vi "GolieKick.vi"(6 "Current State":dbl=4.0, 8 "atacando contra?":bool=TRUE, 9 "balls":T1[](array[typedef])=[{"x"=-974.5169677734375, "y"=-3444.3310546875, "timestamp"=timestamp(2082759045.994995 s since 1904-01-01)}], 10 "Field Size in":T4={"line_width"=10, "field_length"=9000, "field_width"=6000, "boundary_width"=250, "referee_width"=425, "goal_width"=700, "goal_depth"=180, "goal_wall_width"=20, "center_circle_radius"=500, "defense_radius"=500, "defense_stretch"=350, "free_kick_from_defense_dist"=700, "penalty_spot_from_field_line_dist"=450, "penalty_line_from_spot_dist"=350}, 11 "Robot in":T2={"id"=5, "function"=enum."Attacker", "x"=-983.1382446289062, "y"=-3000.010498046875, "orientation"=-1.5516623258590698, "v_tangent"=0.0, "v_normal"=0.0, "v_ang"=0.0, "kick_x"=0.0, "kick_z"=0.0, "dribble"=FALSE, "Timestamp"=timestamp(2082759045.994995 s since 1904-01-01), "dest_x"=0.0, "dest_y"=0.0, "dest_orientation"=0.0, "estimatives"={"est_v_tangent"=0.0, "est_v_normal"=0.0, "est_vx"=0.0, "est_vy"=0.0}}) -> (1 "Next State":dbl=4.0, 2 "Robot out":T2={"id"=5, "function"=enum."Attacker", "x"=-983.1382446289062, "y"=-3000.010498046875, "orientation"=-1.5516623258590698, "v_tangent"=0.0001540345015520423, "v_normal"=0.008599927144915481, "v_ang"=0.002668461263266586, "kick_x"=0.0, "kick_z"=0.0, "dribble"=FALSE, "Timestamp"=timestamp(2082759045.994995 s since 1904-01-01), "dest_x"=0.0, "dest_y"=0.0, "dest_orientation"=0.0, "estimatives"={"est_v_tangent"=0.0, "est_v_normal"=0.0, "est_vx"=0.0, "est_vy"=0.0}})   [LabVIEW 2016]
uses:
  Core/AI Robot.ctl
  Functions Enum.ctl
  Core/Field Size.ctl
  Core/AI Ball.ctl
  <vilib>/Analysis/coordinate.llb/2D Cartesian Coordinate Rotation (Scalar).vi
  <vilib>/Analysis/NI_AALPro.lvlib
panel:
  in  "Longe":dbl=300.0 format="%#_13g"
  out "bola fora?":bool=TRUE
  in  "raio da circunferencia":dbl=175.0 format="%#_13g"
  in  "Cone de rotação":dbl=1.1 format="%#_13g"
  in  "Cone de chute":dbl=0.1 format="%#_13g"
  in  "Perto":dbl=300.0 format="%#_13g"
  in  "min dist to kick":dbl=112.0 format="%#_13g"
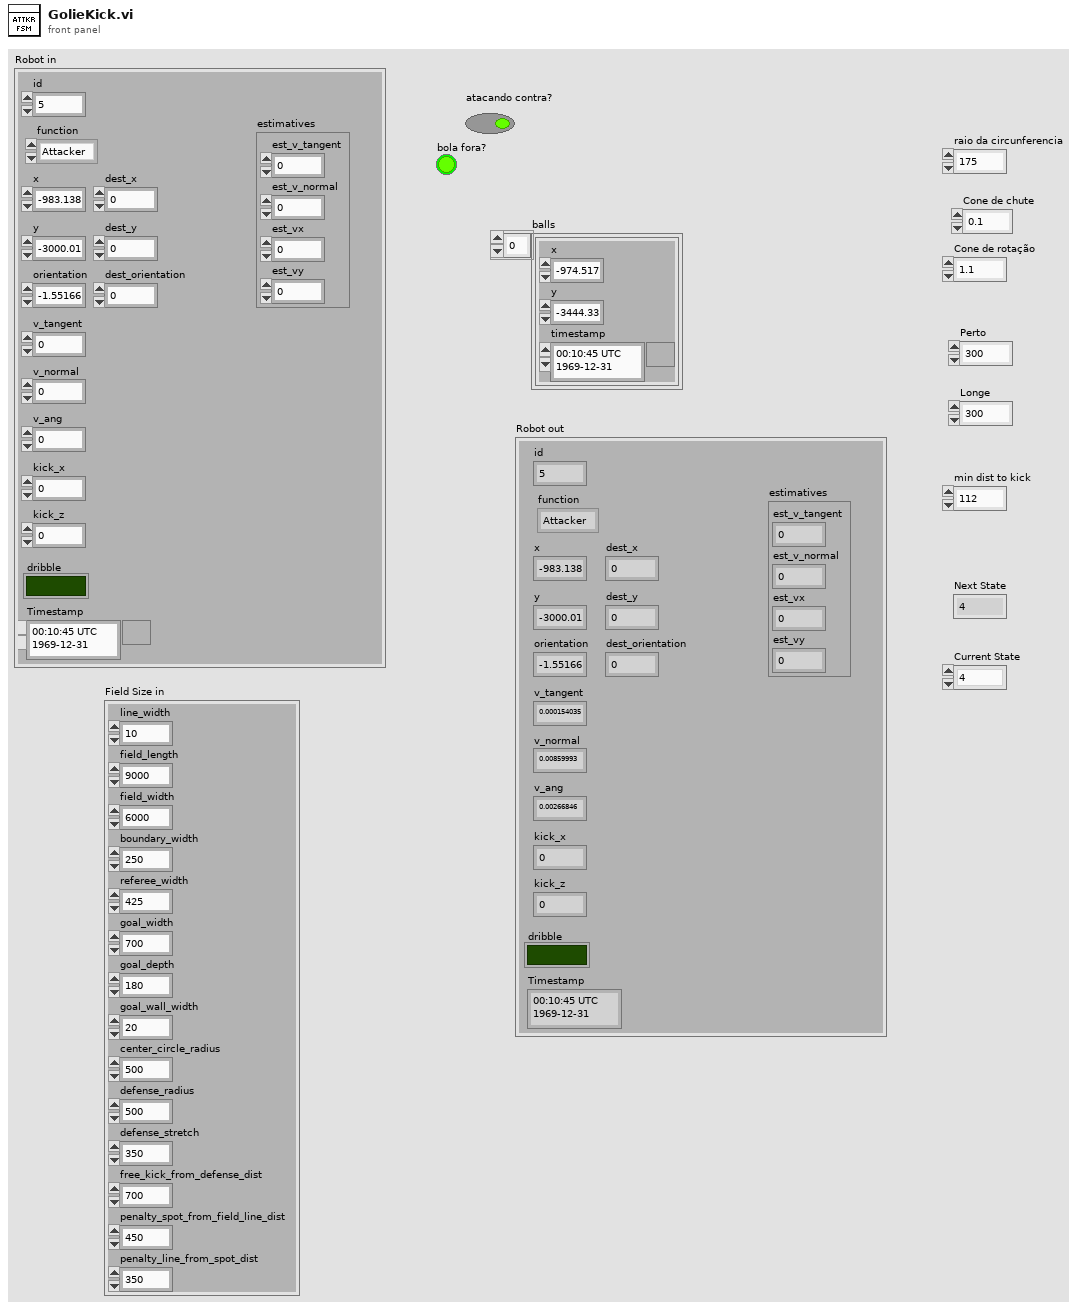
[diagram p1: front panel]
types:
  T1 = typedef "AI Ball.ctl" = cluster{"x":dbl, "y":dbl, "timestamp":timestamp}
  T2 = typedef "AI Robot.ctl" = cluster{"id":u32, "function":T3, "x":dbl, "y":dbl, "orientation":dbl, "v_tangent":dbl, "v_normal":dbl, "v_ang":dbl, "kick_x":dbl, "kick_z":dbl, "dribble":bool, "Timestamp":timestamp, "dest_x":dbl, "dest_y":dbl, "dest_orientation":dbl, "estimatives":cluster{"est_v_tangent":dbl, "est_v_normal":dbl, "est_vx":dbl, "est_vy":dbl}}
  T3 = typedef "Functions Enum.ctl" = enum16{"Attacker", "Goalie", "Defender", "Striker", "Goto 0", "Dummy", "ZigZag"}
  T4 = typedef "Field Size.ctl" = cluster{"line_width":u32, "field_length":u32, "field_width":u32, "boundary_width":u32, "referee_width":u32, "goal_width":u32, "goal_depth":u32, "goal_wall_width":u32, "center_circle_radius":u32, "defense_radius":u32, "defense_stretch":u32, "free_kick_from_defense_dist":u32, "penalty_spot_from_field_line_dist":u32, "penalty_line_from_spot_dist":u32}
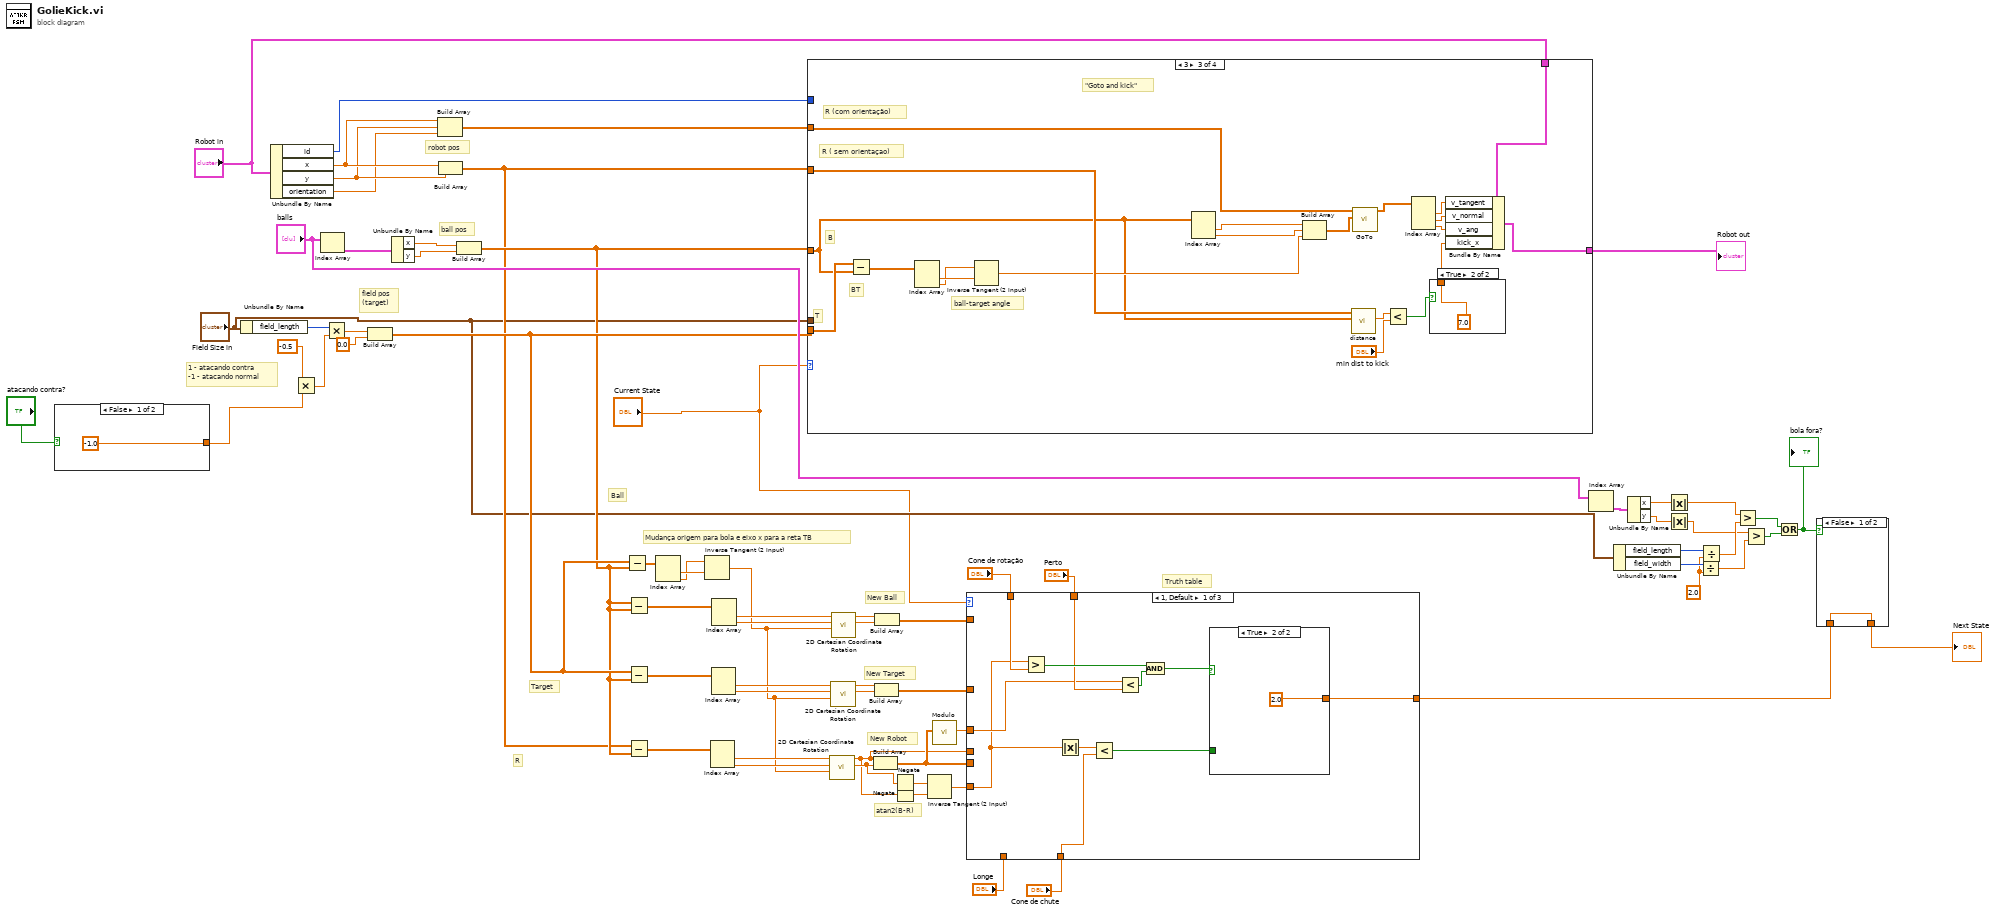
[diagram p0: block diagram]
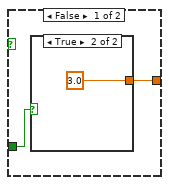
[diagram p2: hidden frame]
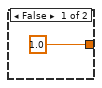
[diagram p3: hidden frame]
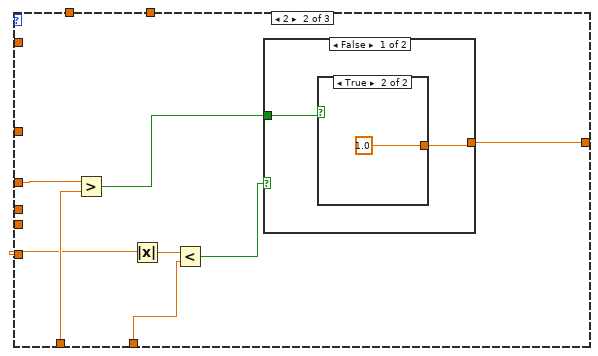
[diagram p4: hidden frame]
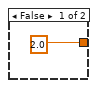
[diagram p5: hidden frame]
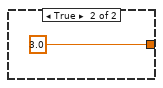
[diagram p6: hidden frame]
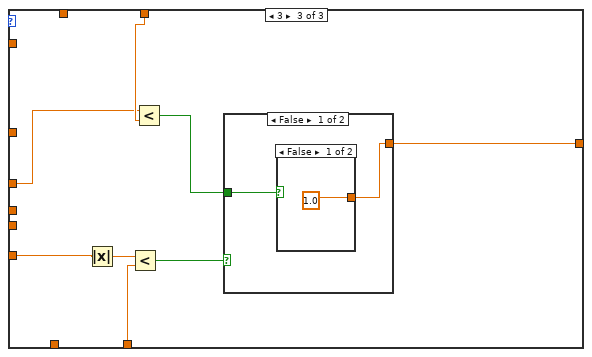
[diagram p7: hidden frame]
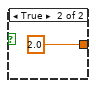
[diagram p8: hidden frame]
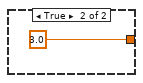
[diagram p9: hidden frame]
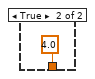
[diagram p10: hidden frame]
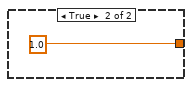
[diagram p11: hidden frame]
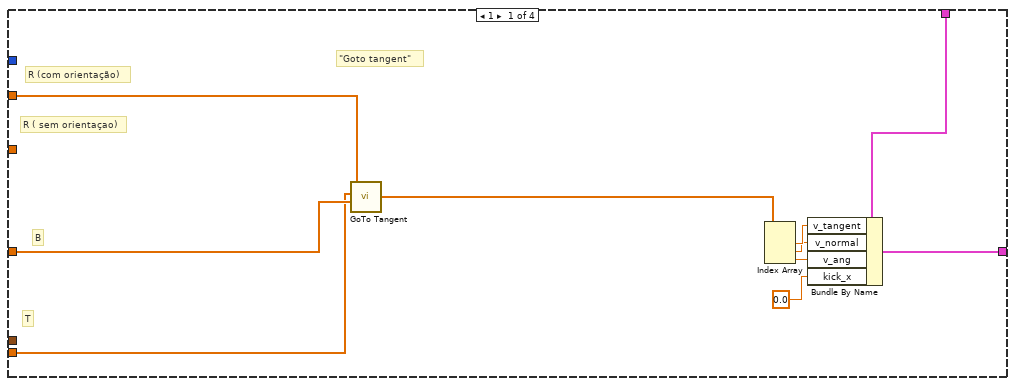
[diagram p12: hidden frame]
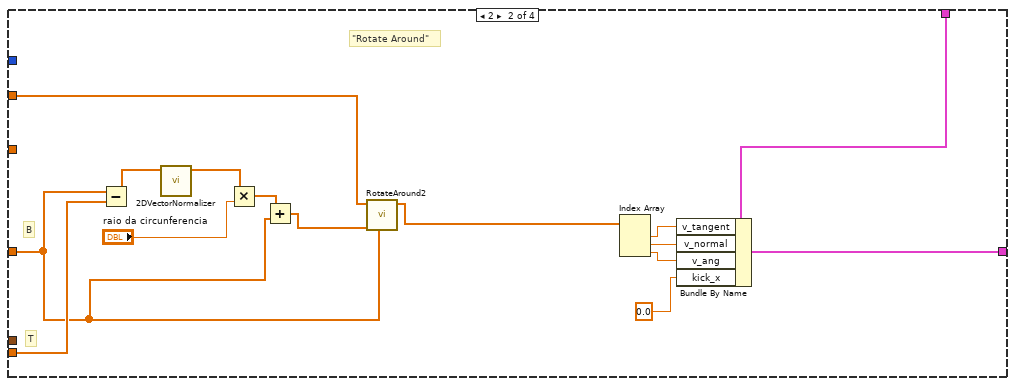
[diagram p13: hidden frame]
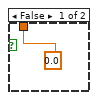
[diagram p14: hidden frame]
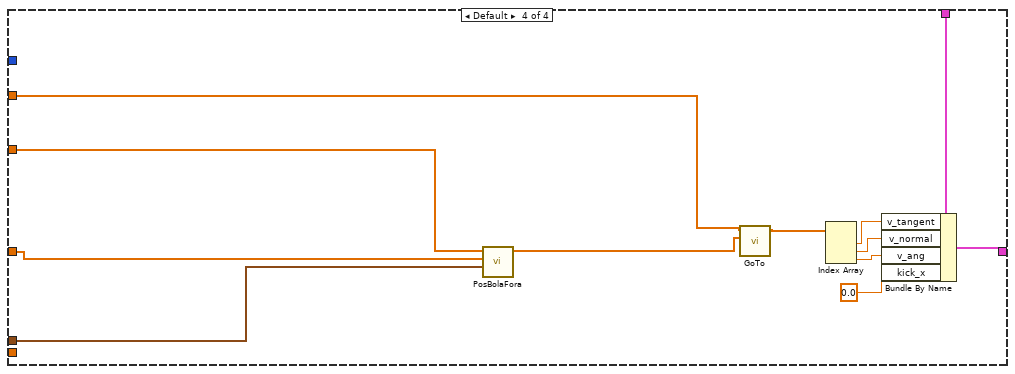
[diagram p15: hidden frame]
diagram:
  w48 = 2.0 ("y")
  # "atan2(B-R)"
  # "New Robot"
  # "New Target"
  # "New Ball"
  # "R"
  # "Ball"
  # "Target"
  # "Mudança origem para bola e eixo x para a reta TB"
  # "1 - atacando contra\n-1 - atacando normal"
  # "Truth table"
  # "robot pos"
  # "field pos\n(target)"
  # "ball pos"
  n1 = case shown="False" "atacando contra?" {
    tunnel: [-1.0 ("attck contra? 2") 1.0] -> w8
    frame False {
    }
    frame True {
    }
  }
  n2 = Unbundle By Name("Field Size in") -> ("field_length"=w67:u32)
  n3 = Unbundle By Name("Robot in") -> ("id"=w1:u32, "x"=w62:dbl, "y"=w61:dbl, "orientation"=w57:dbl)
  n4 = Multiply(x=-0.5, y=w8) -> (x*y=w55:dbl)
  n5 = Index Array(array="balls") -> (element=w68:T1)  [unwired: 1 in]
  n6 = Multiply(x=w67, y=w55) -> (x*y=w66:dbl)
  n7 = Build Array(w66, 0.0 ("element")) -> (w21:dbl[])
  n8 = Unbundle By Name(w68) -> ("x"=w64:dbl, "y"=w63:dbl)
  n9 = Build Array(w62, w61, w57) -> (w59:dbl[])
  n10 = Build Array(w62, w61) -> (w19:dbl[])
  n11 = Build Array(w64, w63) -> (w20:dbl[])
  n12 = Subtract(x=w21, y=w20) -> (x-y=w29:dbl[])
  n13 = Subtract(x=w20, y=w20) -> (x-y=w36:dbl[])
  n14 = Subtract(x=w21, y=w20) -> (x-y=w33:dbl[])
  n15 = Subtract(x=w19, y=w20) -> (x-y=w30:dbl[])
  n16 = Index Array(array=w29) -> (element #1=w28:dbl, element #2=w27:dbl)  [unwired: 2 in]
  n17 = Inverse Tangent (2 Input)(1:w28, 2:w27) -> (0:w22:dbl)
  n18 = Index Array(array=w30) -> (element #1=w32:dbl, element #2=w31:dbl)  [unwired: 2 in]
  n19 = Index Array(array=w33) -> (element #1=w35:dbl, element #2=w34:dbl)  [unwired: 2 in]
  n20 = Index Array(array=w36) -> (element #1=w38:dbl, element #2=w37:dbl)  [unwired: 2 in]
  n21 = case shown="3" "Current State" {
    tunnel: [w80 w95 w116 w130] -> w58
    tunnel: "Robot in" -> [w79 w82 w115 w129]
    tunnel: w59 -> [w77 w94 w100 w121]
    tunnel: w19 -> [_ _ w110 w123]
    tunnel: w20 -> [w73 w81 w96 w124]
    tunnel: w21 -> [w71 w88 w106 _]
    tunnel: "Field Size in" -> [_ _ _ w122]
    tunnel: w1 -> [_ _ _ _]
    frame 1 {
      # "\"Goto tangent\""
      # "B"
      # "T"
      # "R ( sem orientaçao)"
      # "R (com orientação)"
      n22 = call "GoTo Tangent.vi"("Ball"=w73, "Target"=w71, "R"=w77) -> ("Output\nVelocity"=w72:dbl[])  [unwired: 7 in, 1 out]
      n23 = Index Array(array=w72) -> (element #1=w76:dbl, element #2=w75:dbl, element #3=w74:dbl)  [unwired: 3 in]
      n24 = Bundle By Name(cluster=w79, "v_tangent"=w76, "v_normal"=w75, "v_ang"=w74, "kick_x"=0.0) -> (w80:T2)
    }
    frame 2 {
      # "T"
      # "B"
      # "\"Rotate Around\""
      n25 = Subtract(x=w81, y=w88) -> (x-y=w87:dbl[])
      n26 = call "2DVectorNormalizer.vi"("2D vector"=w87) -> ("2D vector 2"=w86:dbl[])  [unwired: 10 in]
      n27 = Multiply(x=w86, y="raio da circunferencia") -> (x*y=w84:dbl[])
      n28 = Add(x=w84, y=w81) -> (x+y=w83:dbl[])
      n29 = call "RotateAround2.vi"("Centre"=w81, "Target"=w83, "Position"=w94) -> ("Output\nVelocity"=w89:dbl[])  [unwired: 8 in]
      n30 = Index Array(array=w89) -> (element #1=w92:dbl, element #2=w91:dbl, element #3=w90:dbl)  [unwired: 3 in]
      n31 = Bundle By Name(cluster=w82, "v_tangent"=w92, "v_normal"=w91, "v_ang"=w90, "kick_x"=0.0) -> (w95:T2)
    }
    frame 3 {
      # "BT"
      # "ball-target angle"
      # "B"
      # "T"
      # "R ( sem orientaçao)"
      # "R (com orientação)"
      # "\"Goto and kick\""
      n32 = Subtract(x=w106, y=w96) -> (x-y=w107:dbl[])
      n33 = Index Array(array=w107) -> (element #1=w109:dbl, element #2=w108:dbl)  [unwired: 2 in]
      n34 = Inverse Tangent (2 Input)(1:w109, 2:w108) -> (0:w105:dbl)
      n35 = Index Array(array=w96) -> (element #1=w104:dbl, element #2=w103:dbl)  [unwired: 2 in]
      n36 = Build Array(w104, w103, w105) -> (w102:dbl[])
      n37 = call "distance.vi"("target pos"=w96, "obj pos"=w110) -> ("sqrt(x)"=w114:dbl)  [unwired: 9 in]
      n38 = call "GoTo.vi"("Target"=w102, "Position"=w100) -> ("Output\nVelocity"=w101:dbl[])  [unwired: 8 in, 1 out]
      n39 = Less?(x=w114, y="min dist to kick") -> (x < y?=w112:bool)
      n40 = Index Array(array=w101) -> (element #1=w99:dbl, element #2=w98:dbl, element #3=w97:dbl)  [unwired: 3 in]
      n41 = case shown="True" w112 {
        tunnel: [0.0 7.0] -> w113
        frame False {
        }
        frame True {
        }
      }
      n42 = Bundle By Name(cluster=w115, "v_tangent"=w99, "v_normal"=w98, "v_ang"=w97, "kick_x"=w113) -> (w116:T2)
    }
    frame Default {
      n43 = call "PosBolaFora.vi"("Field Size in"=w122, "Position da bola"=w124, "Position do robot"=w123) -> ("Target"=w120:dbl[])  [unwired: 8 in]
      n44 = call "GoTo.vi"("Target"=w120, "Position"=w121) -> ("Output\nVelocity"=w119:dbl[])  [unwired: 8 in, 1 out]
      n45 = Index Array(array=w119) -> (element #1=w127:dbl, element #2=w126:dbl, element #3=w125:dbl)  [unwired: 3 in]
      n46 = Bundle By Name(cluster=w129, "v_tangent"=w127, "v_normal"=w126, "v_ang"=w125, "kick_x"=0.0) -> (w130:T2)
    }
  }
  "Robot out" <- w58
  n47 = call-poly <vilib>:"2D Cartesian Coordinate Rotation.vi"("theta"=w22, "y"=w31, "x"=w32) -> ("y out"=w5:dbl, "x out"=w4:dbl)  [unwired: 6 in, 1 out]
  n48 = call-poly <vilib>:"2D Cartesian Coordinate Rotation.vi"("theta"=w22, "y"=w34, "x"=w35) -> ("y out"=w25:dbl, "x out"=w26:dbl)  [unwired: 6 in, 1 out]
  n49 = call-poly <vilib>:"2D Cartesian Coordinate Rotation.vi"("theta"=w22, "y"=w37, "x"=w38) -> ("y out"=w23:dbl, "x out"=w24:dbl)  [unwired: 6 in, 1 out]
  n50 = Build Array(w4, w5) -> (w14:dbl[])
  n51 = Build Array(w26, w25) -> (w15:dbl[])
  n52 = Build Array(w24, w23) -> (w16:dbl[])
  n53 = Negate(x=w5) -> (-x=w7:dbl)
  n54 = Negate(x=w4) -> (-x=w6:dbl)
  n55 = Inverse Tangent (2 Input)(1:w6, 2:w7) -> (0:w12:dbl)
  n56 = call "Modulo.vi"("2D vector"=w14) -> ("Modulo"=w13:dbl)  [unwired: 10 in]
  n57 = case shown="1, Default" "Current State" {
    tunnel: "Longe" -> [_ w153 _]
    tunnel: "Cone de chute" -> [w133 w148 w162]
    tunnel: w16 -> [_ _ _]
    tunnel: w15 -> [_ _ _]
    tunnel: w14 -> [_ _ _]
    tunnel: w13 -> [w137 w154 w165]
    tunnel: w12 -> [w131 w149 w163]
    tunnel: [w135 w152 w167] -> w10
    tunnel: "Cone de rotação" -> [w141 _ _]
    tunnel: "Perto" -> [w138 _ w166]
    tunnel: w4 -> [_ _ _]
    frame 1, Default {
      n58 = Greater?(x=w131, y=w141) -> (0:w140:bool)
      n59 = Absolute Value(x=w131) -> (abs(x)=w134:dbl)
      n60 = Less?(x=w134, y=w133) -> (x < y?=w132:bool)
      n61 = Less?(x=w137, y=w138) -> (x < y?=w139:bool)
      n62 = And(x=w140, y=w139) -> (x .and. y?=w136:bool)
      n63 = case shown="True" w136 {
        tunnel: [w143 2.0] -> w135
        tunnel: w132 -> [w142 _]
        frame False {
          n64 = case shown="True" w142 {
            tunnel: [1.0 3.0] -> w143
            frame False {
            }
            frame True {
            }
          }
        }
        frame True {
        }
      }
    }
    frame 2 {
      n65 = Greater?(x=w154, y=w153) -> (0:w151:bool)
      n66 = Absolute Value(x=w149) -> (abs(x)=w150:dbl)
      n67 = Less?(x=w150, y=w148) -> (x < y?=w147:bool)
      n68 = case shown="False" w147 {
        tunnel: [w155 3.0] -> w152
        tunnel: w151 -> [w156 _]
        frame False {
          n69 = case shown="True" w156 {
            tunnel: [2.0 1.0] -> w155
            frame False {
            }
            frame True {
            }
          }
        }
        frame True {
        }
      }
    }
    frame 3 {
      n70 = Absolute Value(x=w163) -> (abs(x)=w164:dbl)
      n71 = Less?(x=w164, y=w162) -> (x < y?=w161:bool)
      n72 = Less?(x=w165, y=w166) -> (x < y?=w160:bool)
      n73 = case shown="False" w161 {
        tunnel: [w168 3.0] -> w167
        tunnel: w160 -> [w169 _]
        frame False {
          n74 = case shown="False" w169 {
            tunnel: [1.0 2.0] -> w168
            frame False {
            }
            frame True {
            }
          }
        }
        frame True {
        }
      }
    }
  }
  n75 = Index Array(array="balls") -> (element=w53:T1)  [unwired: 1 in]
  n76 = Unbundle By Name("Field Size in") -> ("field_length"=w50:u32, "field_width"=w49:u32)
  n77 = Unbundle By Name(w53) -> ("x"=w52:dbl, "y"=w51:dbl)
  n78 = Absolute Value(x=w52) -> (abs(x)=w47:dbl)
  n79 = Absolute Value(x=w51) -> (abs(x)=w45:dbl)
  n80 = Divide(x=w49, y=w48) -> (x/y=w44:dbl)
  n81 = Divide(x=w50, y=w48) -> (x/y=w46:dbl)
  n82 = Greater?(x=w47, y=w46) -> (0:w43:bool)
  n83 = Greater?(x=w45, y=w44) -> (0:w42:bool)
  n84 = Or(x=w43, y=w42) -> (x .or. y?=w41:bool)
  "bola fora?" <- w41
  n85 = case shown="False" w41 {
    tunnel: [w173 4.0] -> w40
    tunnel: w10 -> [w173 _]
    frame False {
    }
    frame True {
    }
  }
  "Next State" <- w40
